vi "WFGetDtFs.vi"(11 "Waveform":waveform(dbl)) -> (0 "Fs (Hz)":dbl, 3 "dt":dbl)   [LabVIEW 2009]
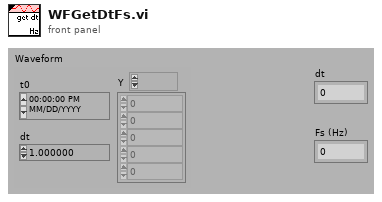
[diagram p1: front panel]
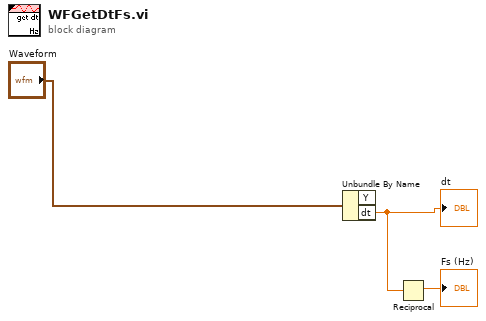
[diagram p0: block diagram]
diagram:
  n1 = Unbundle By Name("Waveform") -> ("dt"=w1:dbl)  [unwired: 1 out]
  "dt" <- w1
  n2 = Reciprocal(x=w1) -> (1/x=→"Fs (Hz)":dbl)
